vi "Log Com.vi"(8 "error in":errorcluster, 9 "Stop Log":bool, 10 "Start Log":bool, 11 "Enum":enum16{"Read", "Write"}(ring)) -> (0 "error out":errorcluster, 1 "Stop Log":bool, 2 "Start Log":bool)   [LabVIEW 2022 SP3]
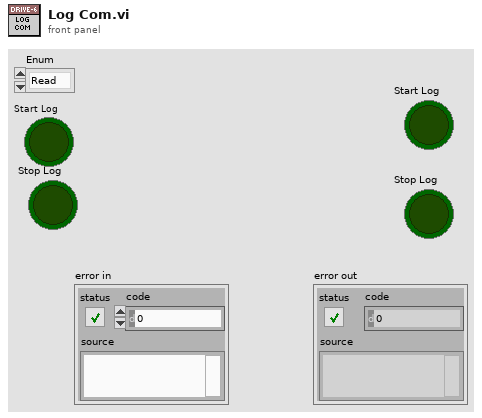
[diagram p1: front panel]
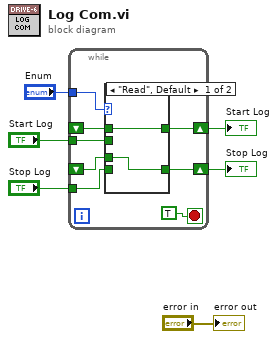
[diagram p0: block diagram]
diagram:
  n1 = while {
    tunnel: "Enum" -> [w14]
    tunnel: "Stop Log" -> [w12]
    shift-right: [w11] -> w3
    shift-left: _ -> [w10]
    tunnel: "Start Log" -> [w9]
    shift-right: [w8] -> w1
    shift-left: _ -> [w7]
    stop <- TRUE stop-if-true
    n2 = case shown="\"Read\", Default" w14 {
      tunnel: w12 -> [_ w18]
      tunnel: [w16 w18] -> w11
      tunnel: w10 -> [w16 _]
      tunnel: w9 -> [_ w17]
      tunnel: [w15 w17] -> w8
      tunnel: w7 -> [w15 _]
      frame "Read", Default {
      }
      frame "Write" {
      }
    }
  }
  "Stop Log" <- w3
  "Start Log" <- w1
  "error out" <- "error in"
